vi "Largest Buffer Size (Plugin).vi"(8 "error in (no error)":errorcluster, 9 "prev engine buffer size (0)":u64 format="%d bytes", 10 "prev string buffer size (0)":u64 format="%d bytes", 11 "Plugin Configuration in":T1={"core"={"name"="", "components"=[], "cycle timing"={"priority"=0, "decimation"=1, "offset"=0}}, "component settings"=[], "threads"=[]}) -> (0 "error out":errorcluster, 1 "largest engine buffer size":u64 format="%d bytes", 2 "largest string buffer size":u64 format="%d bytes", 3 "Plugin Configuration out":T1={"core"={"name"="", "components"=[], "cycle timing"={"priority"=0, "decimation"=1, "offset"=0}}, "component settings"=[], "threads"=[]})   [LabVIEW 2017, in "DSF Core.lvlib" / "Configuration Session.lvclass"]
uses:
  Configuration Session.lvclass
  Typedefs/DSF Direction.ctl
  DSF Core.lvlib
  Typedefs/DSF Timing Info.ctl
  Typedefs/DSF Data Type.ctl
  Typedefs/DSF Settings Info.ctl
  Typedefs/DSF Engine Channel Configuration.ctl
  Typedefs/DSF Engine Transfer Configuration.ctl
  Typedefs/DSF Engine Transfer Group Configuration.ctl
  Typedefs/DSF Engine Plugin Configuration.ctl
  Typedefs/DSF Engine Plugin Thread Configuration.ctl
  Typedefs/DSF Timeout Behavior.ctl
  Typedefs/DSF Version Info.ctl
  Typedefs/DSF Core Channel Configuration.ctl
  Typedefs/DSF Core Transfer Configuration.ctl
  Typedefs/DSF Core Group Configuration.ctl
  Typedefs/DSF Core Thread Configuration.ctl
  Typedefs/DSF Core Plugin Configuration.ctl
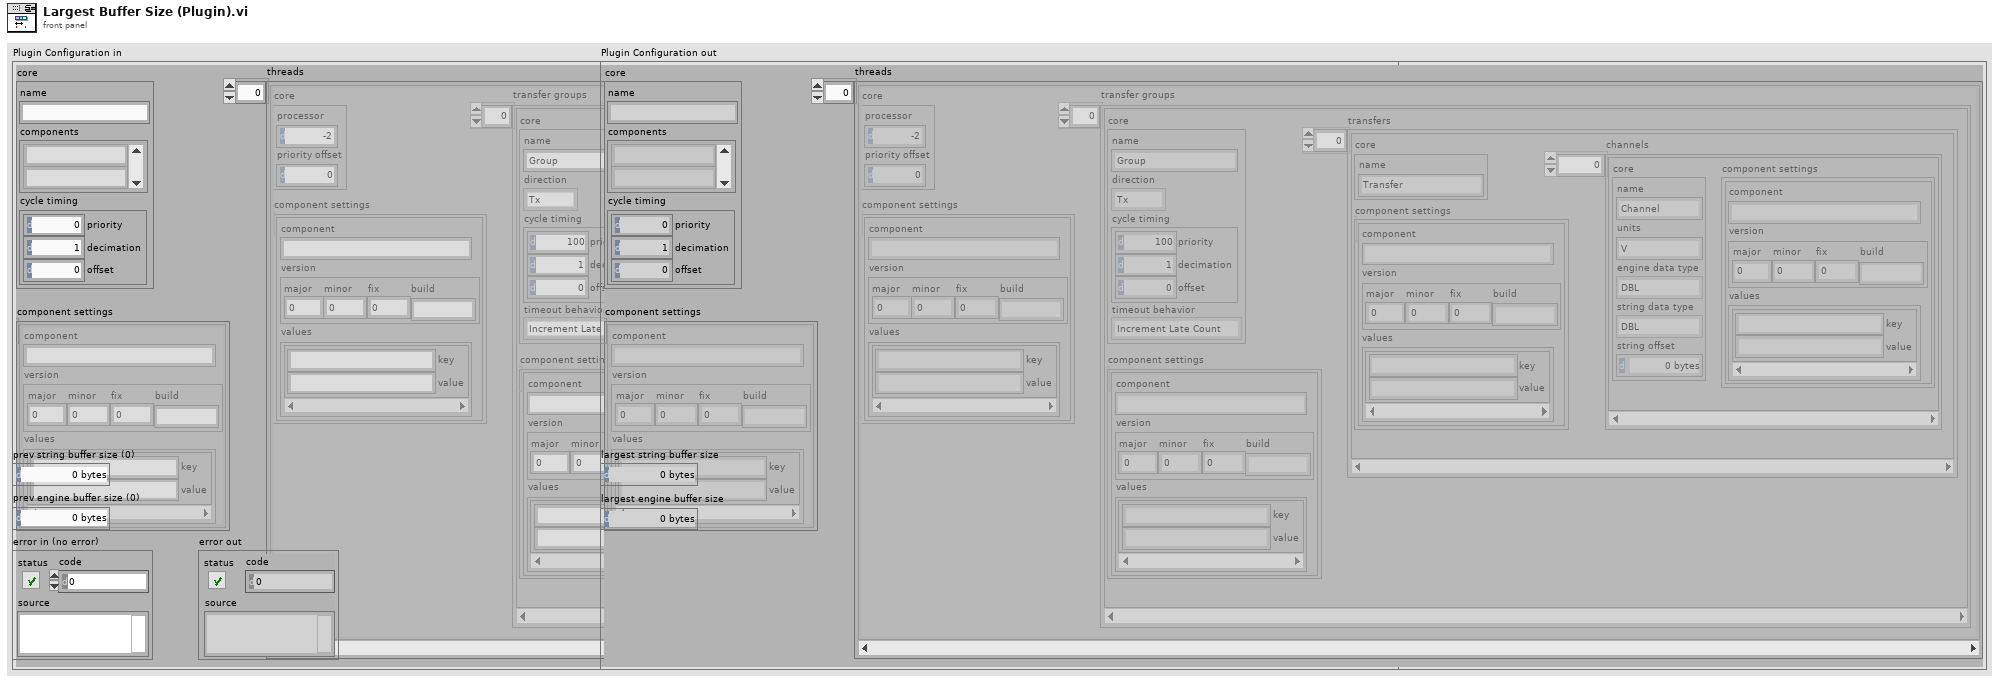
[diagram p1: front panel]
types:
  T1 = typedef "DSF Core.lvlib/DSF Engine Plugin Configuration.ctl" = cluster{"core":T2, "component settings":T4[], "threads":T6[]}
  T2 = typedef "DSF Core.lvlib/DSF Core Plugin Configuration.ctl" = cluster{"name":string, "components":string[], "cycle timing":T3}
  T3 = typedef "DSF Core.lvlib/DSF Timing Info.ctl" = cluster{"priority":u64, "decimation":u64, "offset":u64}
  T4 = typedef "DSF Core.lvlib/DSF Settings Info.ctl" = cluster{"component":string, "version":T5, "values":cluster{"key":string, "value":string}[]}
  T5 = typedef "DSF Core.lvlib/DSF Version Info.ctl" = cluster{"major":u32, "minor":u32, "fix":u32, "build":string}
  T6 = typedef "DSF Core.lvlib/DSF Engine Plugin Thread Configuration.ctl" = cluster{"core":T7, "component settings":T4[], "transfer groups":T8[]}
  T7 = typedef "DSF Core.lvlib/DSF Core Thread Configuration.ctl" = cluster{"processor":i32, "priority offset":i16}
  T8 = typedef "DSF Core.lvlib/DSF Engine Transfer Group Configuration.ctl" = cluster{"core":T9, "component settings":T4[], "transfers":T12[]}
  T9 = typedef "DSF Core.lvlib/DSF Core Group Configuration.ctl" = cluster{"name":string, "direction":T10, "cycle timing":T3, "timeout behavior":T11}
  T10 = typedef "DSF Core.lvlib/DSF Direction.ctl" = enum8{"Tx", "Rx"}
  T11 = typedef "DSF Core.lvlib/DSF Timeout Behavior.ctl" = enum8{"Increment Late Count", "Throw Error"}
  T12 = typedef "DSF Core.lvlib/DSF Engine Transfer Configuration.ctl" = cluster{"core":T13, "component settings":T4[], "channels":T14[]}
  T13 = typedef "DSF Core.lvlib/DSF Core Transfer Configuration.ctl" = cluster{"name":string}
  T14 = typedef "DSF Core.lvlib/DSF Engine Channel Configuration.ctl" = cluster{"core":T15, "component settings":T4[]}
  T15 = typedef "DSF Core.lvlib/DSF Core Channel Configuration.ctl" = cluster{"name":string, "units":string, "engine data type":T16, "string data type":T16, "string offset":u64}
  T16 = typedef "DSF Core.lvlib/DSF Data Type.ctl" = enum8{"Bool", "SGL", "DBL", "I8", "I16", "I32", "I64", "U8", "U16", "U32", "U64"}
  T17 = typedef "DSF Core.lvlib/DSF Engine Transfer Group Configuration.ctl" = cluster{"core":T9, "component settings":T4, "transfers":T12[]}
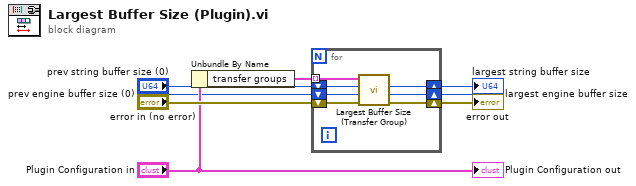
[diagram p0: block diagram]
diagram:
  n1 = Unbundle By Name("Plugin Configuration in") -> ("transfer groups"=w8:T17[])
  n2 = for {
    tunnel: w8 -> [w15] mode=indexing
    shift-right: [w12] -> w3
    shift-left: "prev string buffer size (0)" -> [w10]
    shift-right: [w14] -> w6
    shift-left: "error in (no error)" -> [w13]
    shift-right: [w11] -> w4
    shift-left: "prev engine buffer size (0)" -> [w9]
    n3 = call "Largest Buffer Size (Transfer Group).vi"("error in (no error)"=w13, "prev engine buffer size (0)"=w9, "prev string buffer size (0)"=w10, "Transfer Group Configuration in"=w15) -> ("error out"=w14:errorcluster, "largest engine buffer size"=w11:u64, "largest string buffer size"=w12:u64)  [unwired: 4 in, 1 out]
  }
  "largest string buffer size" <- w3
  "error out" <- w6
  "largest engine buffer size" <- w4
  "Plugin Configuration out" <- "Plugin Configuration in"
